vi "get channels.vi"(11 "Benchmark PID configuration in":refnum<class "Benchmark PID configuration.lvclass">) -> (2 "channels":refnum<class "TBM channel.lvclass">[](array[class]), 3 "Benchmark PID configuration out":refnum<class "Benchmark PID configuration.lvclass">)   [LabVIEW 2018, in "Benchmark PID configuration.lvclass"]
doc: "Returns an array of all Channels currently added to this configuration object."
uses:
  Benchmark PID configuration.lvclass
  <vilib>/NI/Tag Bus Module Framework/channel/TBM channel.lvclass
  Benchmark PID configuration.lvclass/Benchmark PID configuration.ctl
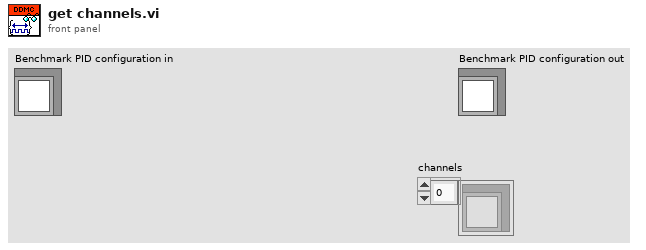
[diagram p1: front panel]
types:
  T1 = typedef "Benchmark PID configuration.lvclass/Line.ctl" = cluster{"PID Name":string, "Setpoint":refnum<class "TBM channel.lvclass">, "Variable":refnum<class "TBM channel.lvclass">, "Output":refnum<class "TBM channel.lvclass">}
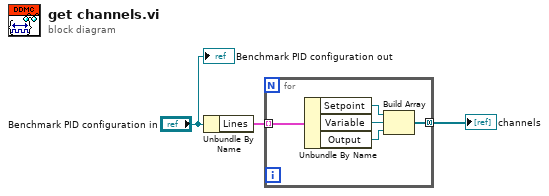
[diagram p0: block diagram]
diagram:
  n1 = Unbundle By Name("Benchmark PID configuration in") -> ("Lines"=w3:T1[])
  n2 = for {
    tunnel: w3 -> [w8] mode=indexing
    tunnel: [w4] -> w2 mode=concatenating
    n3 = Unbundle By Name(w8) -> ("Setpoint"=w7:refnum<class "TBM channel.lvclass">, "Variable"=w5:refnum<class "TBM channel.lvclass">, "Output"=w6:refnum<class "TBM channel.lvclass">)
    n4 = Build Array(w7, w5, w6) -> (w4:refnum<class "TBM channel.lvclass">[])
  }
  "channels" <- w2
  "Benchmark PID configuration out" <- "Benchmark PID configuration in"
